vi "Pre-Purge.vi"(7 "Log File Refnum in":refnum<file>, 8 "error in":errorcluster, 9 "UI Data in":T2, 10 "Handshake Notifier in":refnum<notifier>, 11 "Message Queues in":T1) -> (0 "error out":errorcluster, 1 "UI Data out":T2, 2 "Handshake Notifier out":refnum<notifier>, 3 "Message Queues out":T1, 5 "Log File Refnum out":refnum<file>)   [LabVIEW 2014, in "Controller.lvlib"]
doc: "Clear debris from the boiler ducts."
uses:
  Controller.lvlib
  support/Boiler System Globals.vi
  controls/MHL Status.ctl
  support/Message Queue/Message Cluster.ctl
  support/Message Queue/All Message Queues.ctl
  controls/MHL UI Data.ctl
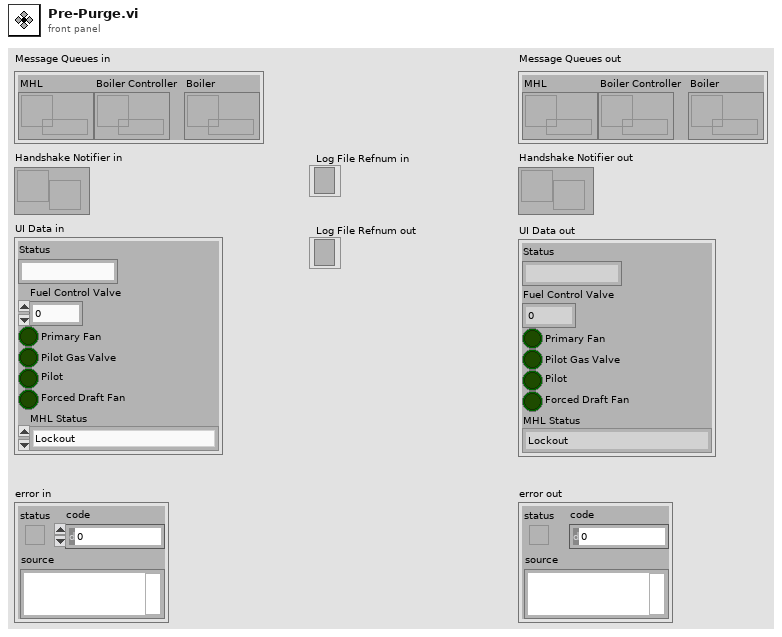
[diagram p1: front panel]
types:
  T1 = typedef "Message Queue.lvlib/All Message Queues.ctl" = cluster{"MHL":refnum<queue>, "Boiler Controller":refnum<queue>, "Boiler":refnum<queue>}
  T2 = typedef "MHL UI Data.ctl" = cluster{"Status":string, "Fuel Control Valve":u32, "Primary Fan":bool, "Pilot Gas Valve":bool, "Pilot":bool, "Forced Draft Fan":bool, "MHL Status":T3}
  T3 = typedef "MHL Status.ctl" = enum16{"Lockout", "Ready", "Pre-Purge", "Pre-Purge Complete", "Pilot On", "Boiler Running", "Shutdown", "Purge"}
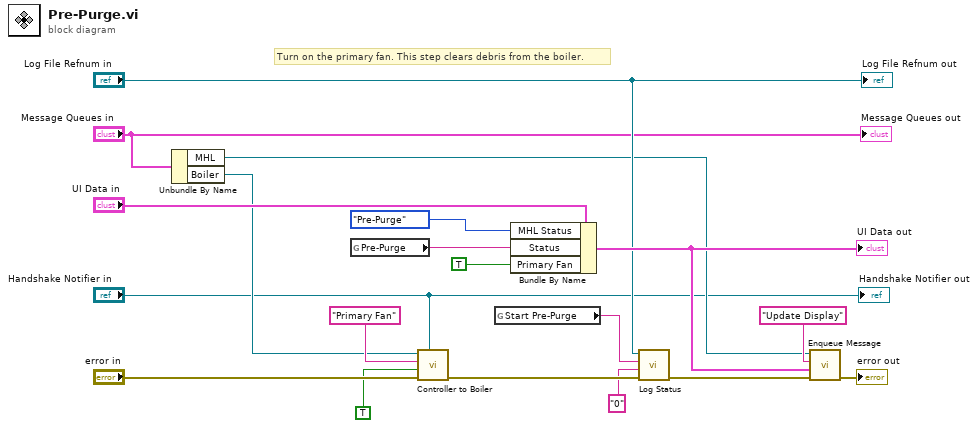
[diagram p0: block diagram]
diagram:
  # "Turn on the primary fan. This step clears debris from the boiler."
  n1 = Unbundle By Name("Message Queues in") -> ("MHL"=w7:refnum<queue>, "Boiler"=w6:refnum<queue>)
  n2 = global read "Boiler System Globals.vi" "Pre-Purge"() -> (w4:string)
  n3 = call "Controller to Boiler.vi"("Notifier"="Handshake Notifier in", "error in"="error in", "Message Data"=TRUE, "Message"="Primary Fan", "Boiler Queue in"=w6) -> ("error out"=w16:errorcluster)  [unwired: 4 in, 2 out]
  n4 = global read "Boiler System Globals.vi" "Start Pre-Purge"() -> (w3:string)
  n5 = Bundle By Name(cluster="UI Data in", "MHL Status"=MHL_Status."Pre-Purge", "Status"=w4, "Primary Fan"=TRUE) -> (w18:T2)
  "UI Data out" <- w18
  n6 = call "Log Status.vi"("error in"=w16, "Event Data String (-)"="0" ("Event Data String"), "Event String"=w3, "Log File Refnum In"="Log File Refnum in") -> ("error out"=w9:errorcluster)  [unwired: 6 in, 1 out]
  n7 = call "Enqueue Message.vi"("error in (no error)"=w9, "Message Data"=w18, "Message"="Update Display", "Message Queue"=w7) -> ("error out"=→"error out":errorcluster)  [unwired: 6 in, 1 out]
  "Log File Refnum out" <- "Log File Refnum in"
  "Message Queues out" <- "Message Queues in"
  "Handshake Notifier out" <- "Handshake Notifier in"
